vi "Destroy Response Session.vi"(8 "error in (no error)":errorcluster, 10 "response":refnum<class "response.lvclass">, 11 "http-client in":refnum<class "http-client.lvclass">) -> (0 "error out":errorcluster, 3 "http-client out":refnum<class "http-client.lvclass">)   [LabVIEW 2020]
uses:
  http-client.lvclass
  response/response.lvclass
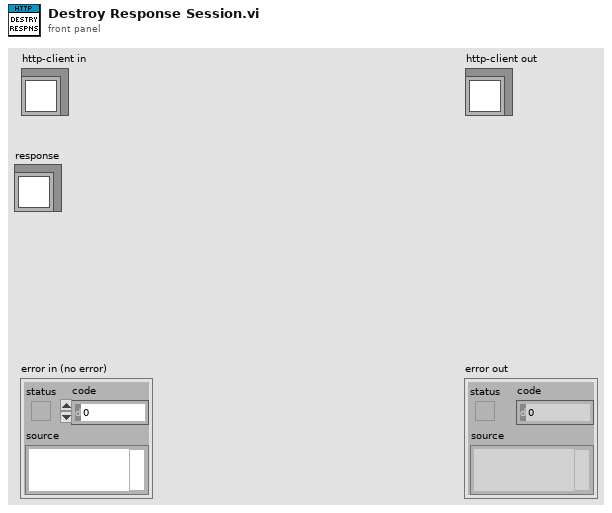
[diagram p1: front panel]
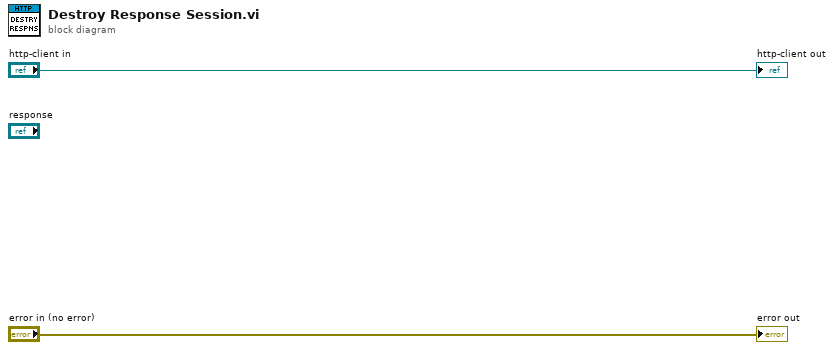
[diagram p0: block diagram]
diagram:
  "error out" <- "error in (no error)"
  "http-client out" <- "http-client in"
